vi "TerminalFactory.vi"(8 "error in":errorcluster, 11 "reference":refnum<vi>) -> (0 "error out":errorcluster, 3 "terminal":refnum<class "Terminal.lvclass">)   [LabVIEW 2014, in "Terminal.lvclass"]
uses:
  Terminal.lvclass
  ControlTerminal/ControlTerminal.lvclass
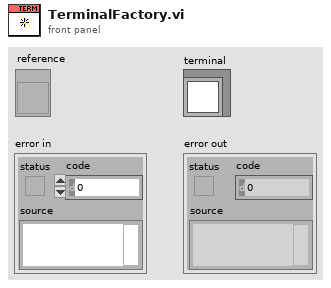
[diagram p1: front panel]
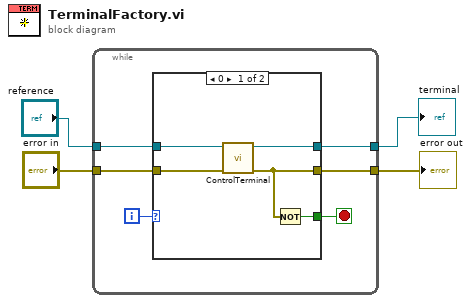
[diagram p0: block diagram]
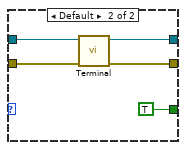
[diagram p2: hidden frame]
diagram:
  n1 = while {
    tunnel: "reference" -> [w9]
    tunnel: "error in" -> [w8]
    tunnel: [w7] -> w2
    tunnel: [w6] -> w1
    i -> [w10]
    stop <- w5 stop-if-true
    n2 = case shown="0" w10 {
      tunnel: w9 -> [w14 w16]
      tunnel: w8 -> [w15 w19]
      tunnel: [w11 w18] -> w7
      tunnel: [w13 w20] -> w6
      tunnel: [w12 TRUE] -> w5
      frame 0 {
        n3 = call "ControlTerminal.vi"("error in"=w15, "reference"=w14) -> ("error out"=w11:errorcluster, "ControlTerminal out"=w13:refnum<class "ControlTerminal.lvclass">)  [unwired: 8 in]
        n4 = Not(x=w11) -> (.not. x?=w12:bool)
      }
      frame Default {
        n5 = call "Terminal.vi"("error in"=w19, "refnum"=w16) -> ("error out"=w18:errorcluster, "terminal"=w20:refnum<class "Terminal.lvclass">)  [unwired: 8 in]
      }
    }
  }
  "error out" <- w2
  "terminal" <- w1
